vi "Setting-CC.vi"(1 "Ctl引用句柄 3":refnum<vi>, 2 "Ctl引用句柄 2":refnum<vi>, 3 "Ctl引用句柄":refnum<vi>, 8 "error in (no error)":errorcluster caption="错误输入（无错误）", 10 "Cluster 2":cluster{"结束温度H":dbl, "变温速率H":dbl}={"结束温度H"=150.0, "变温速率H"=5.0}, 11 "Cluster":T1) -> (0 "error out":errorcluster caption="错误输出")   [LabVIEW 2017]
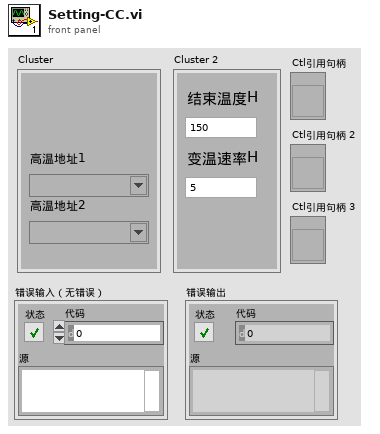
[diagram p1: front panel]
types:
  T1 = cluster{"高温":refnum<visa-resource-name>, "高温 2":refnum<visa-resource-name>}
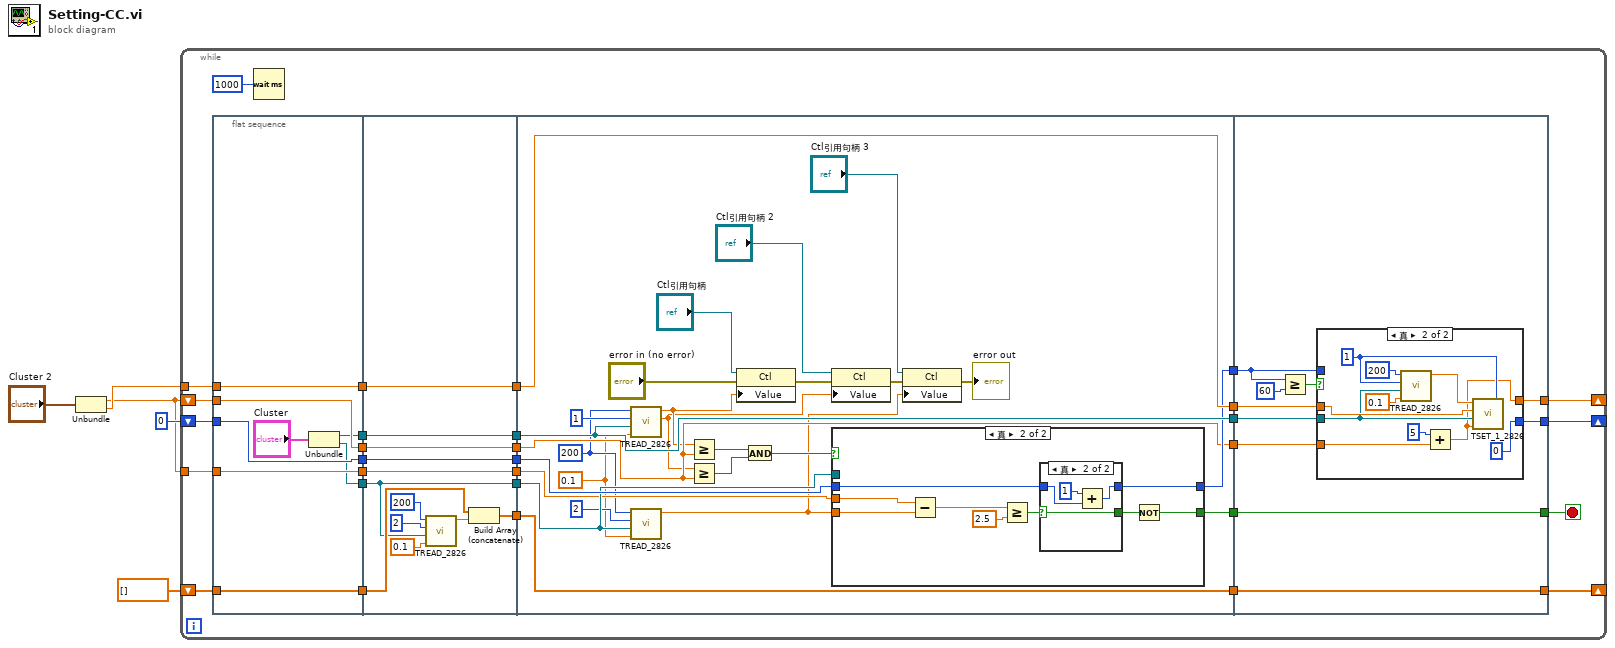
[diagram p0: block diagram]
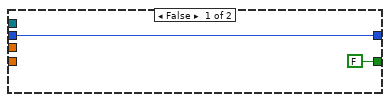
[diagram p2: hidden frame]
diagram:
  n1 = Unbundle("Cluster 2") -> ("结束温度H"=w1:dbl, "变温速率H"=w2:dbl)
  n2 = while {
    shift-right: [w34] -> _
    shift-left: dbl[] [] -> [w35]
    shift-right: [w23] -> _
    shift-left: 0 -> [w29]
    shift-right: [w22] -> _
    shift-left: w1 -> [w19]
    tunnel: w2 -> [w17]
    tunnel: w1 -> [w16]
    stop <- w7 stop-if-true
    n3 = flat-sequence {
      tunnel: w35 -> [w43]
      tunnel: [w43] -> w33
      tunnel: [w36] -> w32
      tunnel: [w37] -> w31
      tunnel: [w41] -> w30
      tunnel: w29 -> [w41]
      tunnel: [w40] -> w20
      tunnel: w19 -> [w40]
      tunnel: [w39] -> w18
      tunnel: w17 -> [w39]
      tunnel: w16 -> [w38]
      tunnel: [w38] -> w15
      tunnel: [w54] -> w14
      tunnel: w33 -> [w55]
      tunnel: w32 -> [w49]
      tunnel: [w50] -> w13
      tunnel: w31 -> [w50]
      tunnel: [w49] -> w12
      tunnel: [w47] -> w11
      tunnel: w30 -> [w47]
      tunnel: [w46] -> w10
      tunnel: w20 -> [w46]
      tunnel: [w45] -> w9
      tunnel: w18 -> [w45]
      tunnel: [w44] -> w8
      tunnel: w15 -> [w44]
      tunnel: w14 -> [w81]
      tunnel: [w81] -> w27
      tunnel: [w75] -> w26
      tunnel: w11 -> [w80]
      tunnel: w12 -> [w79]
      tunnel: w10 -> [w74]
      tunnel: [w78] -> w25
      tunnel: w9 -> [w78]
      tunnel: [w77] -> w24
      tunnel: w13 -> [w77]
      tunnel: [w74] -> w21
      tunnel: w8 -> [w70]
      tunnel: [w66] -> w6
      tunnel: w27 -> [w108]
      tunnel: w26 -> [w104]
      tunnel: w25 -> [w103]
      tunnel: w24 -> [w102]
      tunnel: w21 -> [w100]
      tunnel: [w108] -> w34
      tunnel: [w105] -> w23
      tunnel: [w101] -> w22
      tunnel: [w99] -> w7
      tunnel: w6 -> [w99]
      frame #0 {
        n4 = Unbundle("Cluster") -> ("高温"=w37:refnum<visa-resource-name>, "高温 2"=w36:refnum<visa-resource-name>)
      }
      frame #1 {
        n5 = call "TREAD_2826.vi"("Unknown Param 2"=0.1, "VISA resource name"=w49, "Address No."=i8 2, "Unknown Param"=200) -> ("PV"=w48:dbl)  [unwired: 3 out]
        n6 = Build Array (concatenate)(w55, w48) -> (w54:dbl[])
      }
      frame #2 {
        w67 = 0.1
        w68 = 200
        n7 = call "TREAD_2826.vi"("Unknown Param 2"=w67, "VISA resource name"=w77, "Address No."=i8 1, "Unknown Param"=w68) -> ("SV"=w57:dbl, "PV"=w58:dbl)  [unwired: 2 out]
        n8 = call "TREAD_2826.vi"("Unknown Param 2"=w67, "VISA resource name"=w79, "Address No."=i8 2, "Unknown Param"=w68) -> ("PV"=w56:dbl)  [unwired: 3 out]
        n9 = Greater Or Equal?(x=w58, y=w74) -> (x >= y?=w72:bool)
        n10 = Greater Or Equal?(x=w57, y=w74) -> (x >= y?=w71:bool)
        n11 = property class="Ctl"(reference="Ctl引用句柄", error in="error in (no error)", "Value"=w58) -> (error out=w65:errorcluster)  [unwired: 1 out]
        n12 = And(x=w72, y=w71) -> (x .and. y?=w73:bool)
        n13 = property class="Ctl"(reference="Ctl引用句柄 2", error in=w65, "Value"=w57) -> (error out=w64:errorcluster)  [unwired: 1 out]
        n14 = case shown="真" w73 {
          tunnel: w80 -> [w83 w92]
          tunnel: [w83 w91] -> w75
          tunnel: w79 -> [_ _]
          tunnel: w70 -> [_ w88]
          tunnel: w56 -> [_ w87]
          tunnel: [FALSE w85] -> w66
          frame False {
          }
          frame True {
            n15 = Subtract(x=w88, y=w87) -> (x-y=w90:dbl)
            n16 = Greater Or Equal?(x=w90, y=2.5) -> (x >= y?=w86:bool)
            n17 = case shown="真" w86 {
              selector: w86 -> [w93 w95]
              tunnel: [w94 w97] -> w91
              tunnel: w92 -> [w94 w96]
              tunnel: [w93 w95] -> w84
              frame False {
              }
              frame True {
                n18 = Add(x=1, y=w96) -> (x+y=w97:i32)
              }
            }
            n19 = Not(x=w84) -> (.not. x?=w85:bool)
          }
        }
        n20 = property class="Ctl"(reference="Ctl引用句柄 3", error in=w64, "Value"=w56) -> (error out=→"error out":errorcluster)  [unwired: 1 out]
      }
      frame #3 {
        n21 = Greater Or Equal?(x=w104, y=60) -> (x >= y?=w106:bool)
        n22 = case shown="真" w106 {
          tunnel: [w110 w111] -> w101
          tunnel: w100 -> [w110 w118]
          tunnel: [w109 0] -> w105
          tunnel: w104 -> [w109 _]
          tunnel: w103 -> [_ w115]
          tunnel: w102 -> [_ w114]
          frame False {
          }
          frame True {
            w113 = i8 1 ("Address No.")
            n23 = call "TREAD_2826.vi"("Unknown Param 2"=0.1, "VISA resource name"=w114, "Address No."=w113, "Unknown Param"=200) -> ("PV"=w112:dbl)  [unwired: 3 out]
            n24 = Add(x=5, y=w118) -> (x+y=w111:dbl)
            n25 = call "TSET_1_2826.vi"("Address No."=w113, "T-Ending, C"=w111, "VISA resource name"=w114, "cooling/heating rate, C/min"=w115, "T-Starting, C"=w112) -> ()
          }
        }
      }
    }
    n26 = Wait (ms)(milliseconds to wait=1000) -> ()  [unwired: 1 out]
  }
